vi "Num Rep to String.vi"(3 "Rep":T1) -> (1 "String":string)   [LabVIEW 2023, in "VIDoc Parsing.lvlib"]
uses:
  VIDoc Parsing.lvlib
  <vilib>/numeric/LVNumericRepresentation.ctl
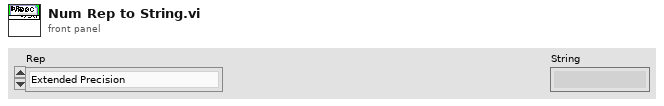
[diagram p1: front panel]
types:
  T1 = typedef "LVNumericRepresentation.ctl" = enum32{"Extended Precision", "Double Precision", "Single Precision", "Long", "Word", "Byte", "Unsigned Long", "Unsigned Word", "Unsigned Byte", "Complex Extended", "Complex Double", "Complex Single", "Quad", "Unsigned Quad", "Fixed-Point"}
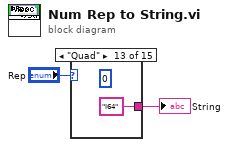
[diagram p0: block diagram]
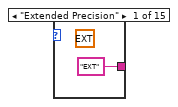
[diagram p2: hidden frame]
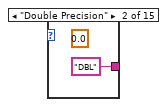
[diagram p3: hidden frame]
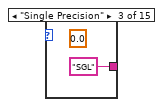
[diagram p4: hidden frame]
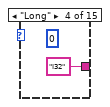
[diagram p5: hidden frame]
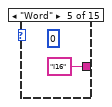
[diagram p6: hidden frame]
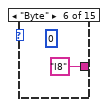
[diagram p7: hidden frame]
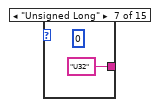
[diagram p8: hidden frame]
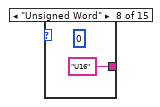
[diagram p9: hidden frame]
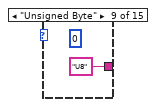
[diagram p10: hidden frame]
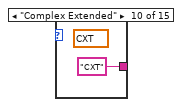
[diagram p11: hidden frame]
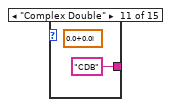
[diagram p12: hidden frame]
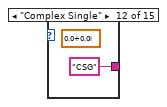
[diagram p13: hidden frame]
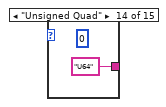
[diagram p14: hidden frame]
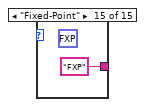
[diagram p15: hidden frame]
diagram:
  n1 = case shown="\"Quad\"" "Rep" {
    tunnel: ["EXT" "DBL" "SGL" "I32" "I16" "I8" "U32" "U16" "U8" "CXT" "CDB" "CSG" "I64" "U64" "FXP"] -> w1
    frame "Extended Precision" {
      (unwired) ext 0.0
    }
    frame "Double Precision" {
      (unwired) 0.0
    }
    frame "Single Precision" {
      (unwired) sgl 0.0
    }
    frame "Long" {
      (unwired) 0
    }
    frame "Word" {
      (unwired) i16 0
    }
    frame "Byte" {
      (unwired) i8 0
    }
    frame "Unsigned Long" {
      (unwired) u32 0
    }
    frame "Unsigned Word" {
      (unwired) u16 0
    }
    frame "Unsigned Byte" {
      (unwired) u8 0
    }
    frame "Complex Extended" {
      (unwired) cxt 0.0+0.0i
    }
    frame "Complex Double" {
      (unwired) cdb 0.0+0.0i
    }
    frame "Complex Single" {
      (unwired) csg 0.0+0.0i
    }
    frame "Quad" {
      (unwired) i64 0
    }
    frame "Unsigned Quad" {
      (unwired) u64 0
    }
    frame "Fixed-Point" {
      (unwired) fxp<+,1,1> 0.0
    }
  }
  "String" <- w1
